vi "本地网络变量读写.vi"() -> ()   [LabVIEW 2016]
panel:
  out "数组 2":timestamp[](array[timestamp])
  out "数组":cluster{"IP":string, "port":i32}[][](array[cluster])
  out "引用句柄数组输出":refnum<k21>[](array[refnum])
  out "本地PSP根变量容器":refnum<k21>
  out "元素":refnum<k21>
  in  "共享变量引用句柄输入":refnum<k21>
  out "错误输出":errorcluster
  in  "错误输入（无错误）":errorcluster
  in  "停止":bool
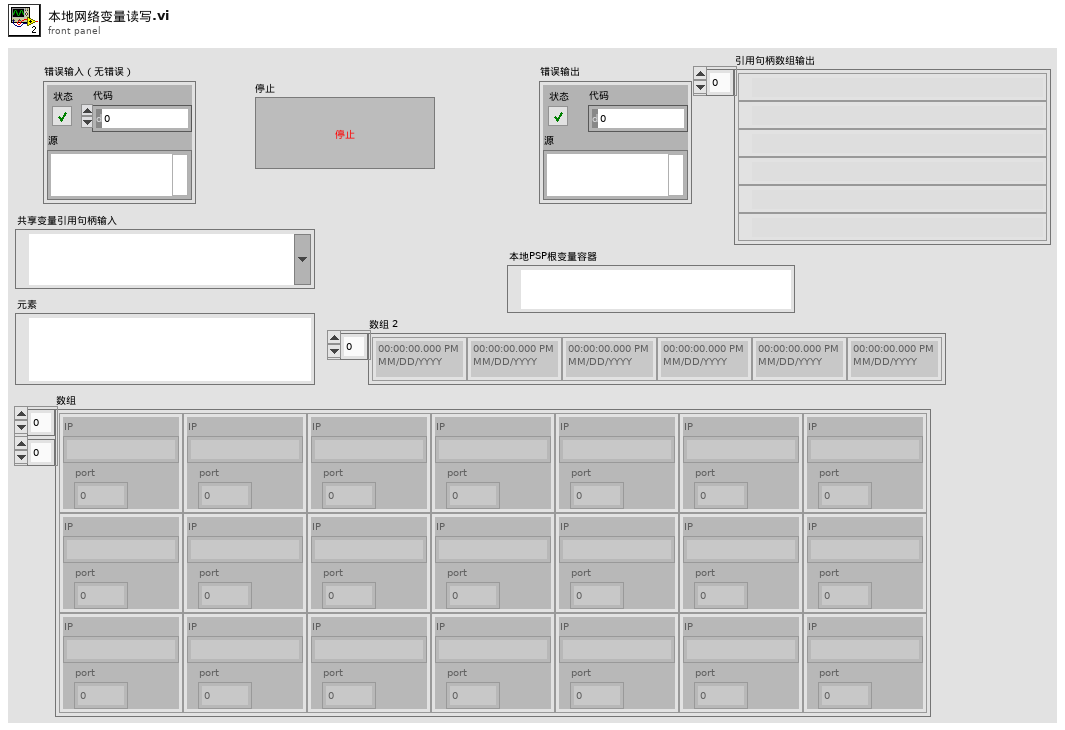
[diagram p1: front panel]
types:
  T1 = cluster{"Read Access":enum8{"Allowed", "Required", "Denied"}, "Write Access":enum8{"Allowed", "Required", "Denied"}}
  T2 = cluster{"Read Access":enum8{"Allowed", "Required", "None"}, "Write Access":enum8{"Allowed", "Required", "None"}}
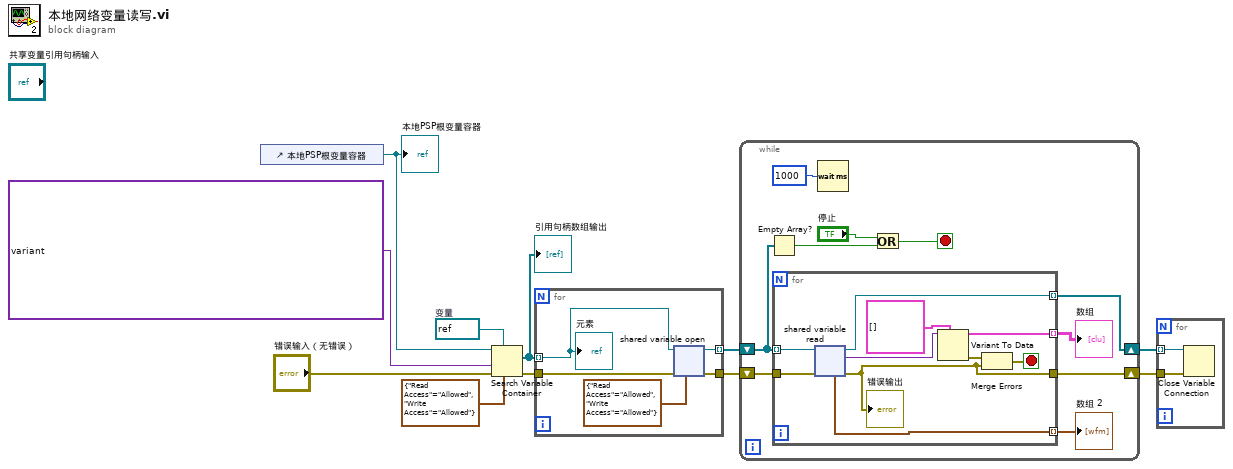
[diagram p0: block diagram]
diagram:
  w10 = refnum<k21> refnum  # 变量
  n1 = control-ref of="本地PSP根变量容器"() -> (w8:refnum<k21>)
  "本地PSP根变量容器" <- w8
  n2 = Search Variable Container(6:T1 {"Read Access"=enum."Allowed", "Write Access"=enum."Allowed"} ("访问类型"), 7:w10, 8:"错误输入（无错误）", 9:variant(cluster{"IP":string, "port":i32}[] []) ("变体"), 11:w8) -> (0:w5:errorcluster, 2:w6:refnum<k21>[])  [unwired: 1 in, 1 out]
  "引用句柄数组输出" <- w6
  n3 = for {
    tunnel: w6 -> [w14] mode=indexing
    tunnel: w5 -> [w15]
    tunnel: [w13] -> w4 mode=indexing
    tunnel: [w12] -> w3
    n4 = shared-variable-open(w14, w15, T2 {"Read Access"=enum."Allowed", "Write Access"=enum."Allowed"} ("权限")) -> (w13:refnum<k21>, w12:errorcluster)
    "元素" <- w14
  }
  n5 = while {
    shift-right: [w25] -> w2
    shift-left: w4 -> [w17]
    shift-right: [w24] -> w1
    shift-left: w3 -> [w26]
    stop <- w19 stop-if-true
    n6 = Empty Array?(array=w17) -> (empty?=w18:bool)
    n7 = for {
      tunnel: [w36] -> w25 mode=indexing
      tunnel: [w31] -> w24
      tunnel: w17 -> [w33] mode=indexing
      tunnel: w26 -> [w32]
      tunnel: [w30] -> w21 mode=indexing
      tunnel: [w29] -> w20 mode=indexing
      stop <- w28 stop-if-true
      n8 = shared-variable-read(w33, w32) -> (w36:refnum<k21>, w31:errorcluster, w35:variant, w29:timestamp)
      "错误输出" <- w31
      n9 = Variant To Data(type=cluster{"IP":string, "port":i32}[] [] ("数组"), Variant=w35) -> (data=w30:cluster{"IP":string, "port":i32}[], error out=w27:errorcluster)  [unwired: 1 in]
      n10 = Merge Errors(w27, w31) -> (w28:errorcluster)
    }
    "数组" <- w21
    "数组 2" <- w20
    n11 = Wait (ms)(milliseconds to wait=u32 1000 ("等待时间（毫秒）")) -> ()  [unwired: 1 out]
    n12 = Or(x="停止", y=w18) -> (x .or. y?=w19:bool)
  }
  n13 = for {
    tunnel: w2 -> [w38] mode=indexing
    tunnel: w1 -> [w37]
    n14 = Close Variable Connection(8:w37, 11:w38) -> ()  [unwired: 1 out]
  }
